vi "CU_CorrelationCoeffs.vi"(10 "Signal X":waveform(dbl), 11 "Signal Y (Array)":waveform(dbl)[](array[waveform])) -> (3 "CorrCoefficients":dbl[](array[numeric]))   [LabVIEW 2016, in "Classifier.lvlib"]
uses:
  4. Accuracy Assessment for EEG Classification/Classifier.lvlib
  <vilib>/gmath/NI_Gmath.lvlib
panel:
  # "This VI is a part of BCI Design library, http://www.ru-bci.org \nCopyright © 2020, Sotnikov Peter, All rights reserved. License: GNU GPLv3"
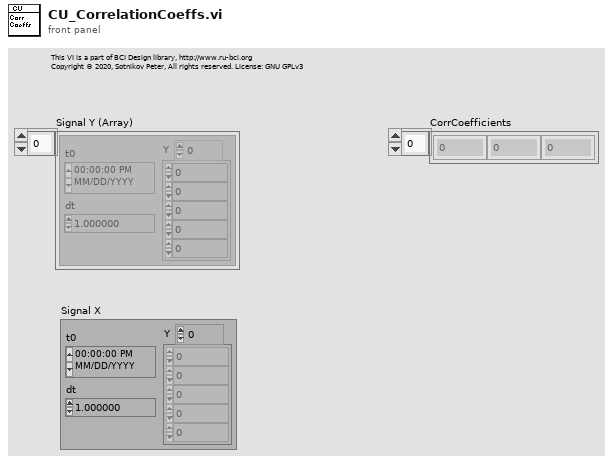
[diagram p1: front panel]
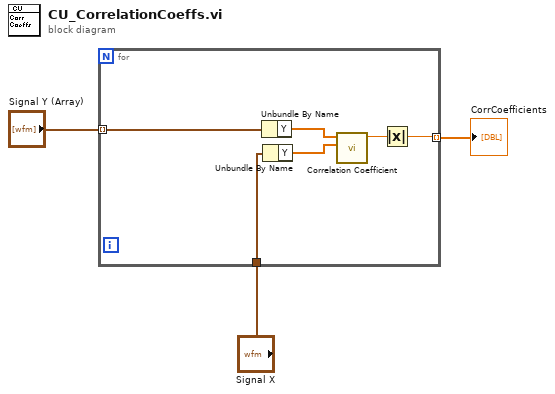
[diagram p0: block diagram]
diagram:
  n1 = for {
    tunnel: "Signal Y (Array)" -> [w4] mode=indexing
    tunnel: "Signal X" -> [w9]
    tunnel: [w5] -> w1 mode=indexing
    n2 = Unbundle By Name(w4) -> ("Y"=w8:dbl[])
    n3 = Unbundle By Name(w9) -> ("Y"=w7:dbl[])
    n4 = call <vilib>:"Correlation Coefficient.vi"("Y"=w7, "X"=w8) -> ("correlation coefficient r"=w6:dbl)  [unwired: 8 in, 1 out]
    n5 = Absolute Value(x=w6) -> (abs(x)=w5:dbl)
  }
  "CorrCoefficients" <- w1
